vi "Shutdown Daemon.vi"(8 "error in":errorcluster, 11 "TCP slave in":refnum<class "TCP Slave.lvclass">) -> (0 "error out":errorcluster)   [LabVIEW 2021, in "TCP Slave.lvclass"]
doc: "Sends a notification to the daemon and connection handlers, commanding them to quit."
uses:
  TCP Slave.lvclass
  TCP Slave.lvclass/TCP Slave.ctl
  Network Slave.lvclass
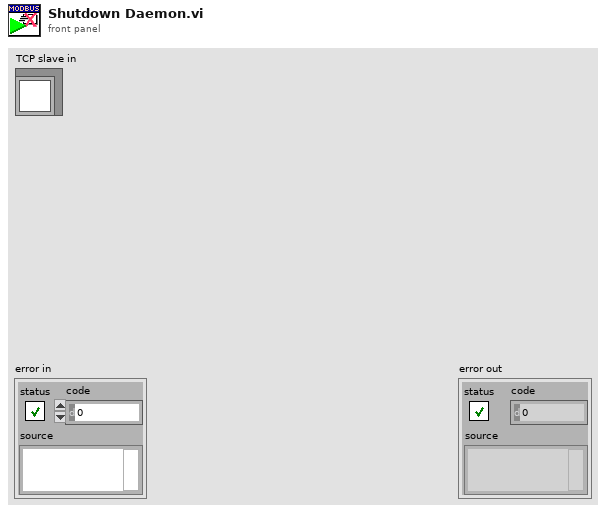
[diagram p1: front panel]
types:
  T1 = typedef "TCP Slave.lvclass/Connection Counter.ctl" = cluster{"Currently Connected":u32, "Connection Records":refnum<data-value>[]}
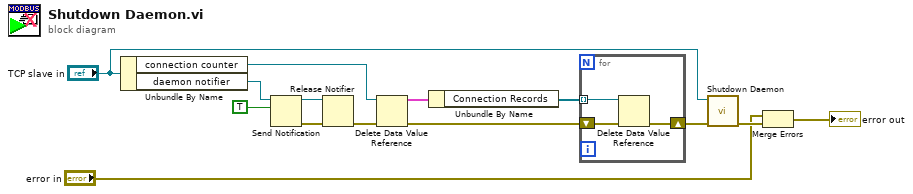
[diagram p0: block diagram]
diagram:
  n1 = Unbundle By Name("TCP slave in") -> ("connection counter"=w7:refnum<data-value>, "daemon notifier"=w11:refnum<notifier>)
  n2 = Send Notification(notification=TRUE, notifier=w11) -> (notifier out=w13:refnum<notifier>, error out=w12:errorcluster)  [unwired: 1 in]
  n3 = Release Notifier(notifier=w13, error in (no error)=w12) -> (error out=w8:errorcluster)  [unwired: 1 in, 2 out]
  n4 = Delete Data Value Reference(data value reference=w7, error in=w8) -> (data value=w4:T1, error out=w6:errorcluster)
  n5 = Unbundle By Name(w4) -> ("Connection Records"=w3:refnum<data-value>[])
  n6 = for {
    shift-right: [w15] -> w5
    shift-left: w6 -> [w16]
    tunnel: w3 -> [w17] mode=indexing
    n7 = Delete Data Value Reference(data value reference=w17, error in=w16) -> (error out=w15:errorcluster)  [unwired: 1 out]
  }
  n8 = call-parent "Shutdown Daemon.vi"("error in"=w5, "network slave in"="TCP slave in") -> ("error out"=w10:errorcluster)  [unwired: 9 in]
  n9 = Merge Errors("error in", w10) -> (→"error out":errorcluster)
